vi "Patch data preview-Obtain single cycle data.vi"(9 "Channel to load":enum16{"Red", "Green"}(ring), 10 "Global cycle number among all trials":i32, 11 "Register cluster":T1) -> (0 "error out":errorcluster, 3 "Data from single channel single cycle":dbl[](array[numeric]), 5 "Double channel data":dbl[][](array[numeric]))   [LabVIEW 2020]
uses:
  Typedefs/Patch viewer internal cluster.ctl
  <vilib>/vision/Image Controls.llb/IMAQ Image.ctl
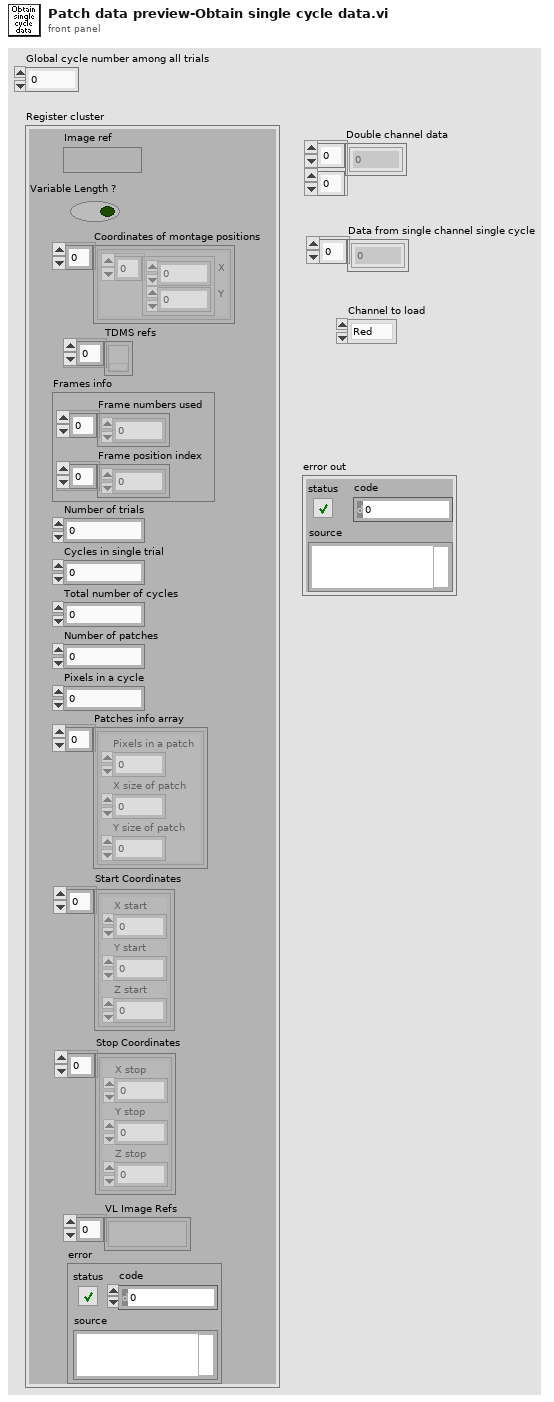
[diagram p1: front panel]
types:
  T1 = typedef "Patch viewer internal cluster.ctl" = cluster{"Image ref":T2, "Variable Length ?":bool, "Coordinates of montage positions":cluster{"X\n\nY":i32[]}[], "TDMS refs":refnum<k34>[], "Frames info":cluster{"Frame numbers used":i32[], "Frame position index":i32[]}, "Number of trials":i32, "Cycles in single trial":i32, "Total number of cycles":i32, "Number of patches":i32, "Pixels in a cycle":i32, "Patches info array":cluster{"Pixels in a patch":i32, "X size of patch":i32, "Y size of patch":i32}[], "Start Coordinates":cluster{"X start":i32, "Y start":i32, "Z start":i32}[], "Stop Coordinates":cluster{"X stop":i32, "Y stop":i32, "Z stop":i32}[], "VL Image Refs":T2[], "error":errorcluster}
  T2 = typedef "IMAQ Image.ctl" = refnum<image>
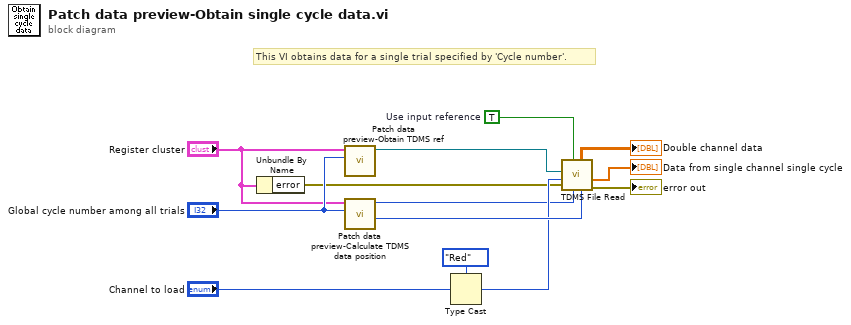
[diagram p0: block diagram]
diagram:
  w2 = TRUE  # Use input reference
  # "This VI obtains data for a single trial specified by 'Cycle number'."
  n1 = Unbundle By Name("Register cluster") -> ("error"=w7:errorcluster)
  n2 = call "Patch data preview-Obtain TDMS ref.vi"("Cycle number"="Global cycle number among all trials", "Register cluster"="Register cluster") -> ("TDMS ref"=w5:refnum<k34>)  [unwired: 8 in, 1 out]
  n3 = call "Patch data preview-Calculate TDMS data position.vi"("Global cycle number among all trials"="Global cycle number among all trials", "Register cluster"="Register cluster") -> ("Cycle's data length"=w13:i64, "Cycle's data start index in current trial"=w3:i64)  [unwired: 8 in]
  n4 = Type Cast(type=enum16{"Red", "Green", "Both"}."Red" ("Channel to load"), x="Channel to load") -> (*(type *) &x=w9:enum16{"Red", "Green", "Both"})
  n5 = call "TDMS File Read.vi"("count (-1: all)"=w13, "offset (0)"=w3, "Use input reference (F)"=w2, "Error In"=w7, "Channel to load"=w9, "tdms file ref"=w5) -> ("Error Out"=→"error out":errorcluster, "Single channel data"=→"Data from single channel single cycle":dbl[], "Double channel data"=→"Double channel data":dbl[][])  [unwired: 1 in, 2 out]
